vi "simulation_to_image.vi"() -> (3 "Image Out":T1)   [LabVIEW 2010]
uses:
  <vilib>/vision/Image Controls.llb/IMAQ Image.ctl
  simulation_globals.vi
  red_tweezers_globals_INTERNAL.vi
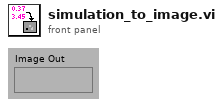
[diagram p1: front panel]
types:
  T1 = typedef "IMAQ Image.ctl" = refnum<image>
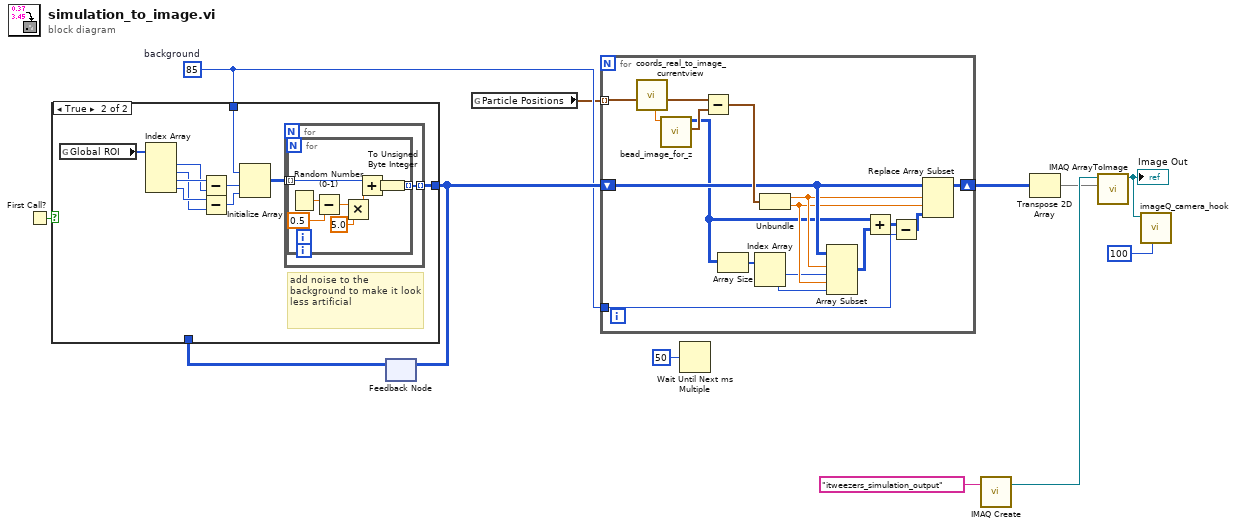
[diagram p0: block diagram]
diagram:
  w7 = u8 85  # background
  n1 = First Call?() -> (First Call?: T/F=w9:bool)
  n2 = feedback #1() -> (w10:u8[][])  [unwired: 1 in]
  n3 = case shown="True" w9 {
    tunnel: [w13 w15] -> w8
    tunnel: w10 -> [w13 _]
    tunnel: w7 -> [_ w14]
    frame False {
    }
    frame True {
      # "add noise to the background to make it look less artificial"
      n4 = global read "red_tweezers_globals_INTERNAL.vi" "Global ROI"() -> (w23:i32[])
      n5 = Index Array(array=w23) -> (element #1=w21:i32, element #2=w19:i32, element #3=w22:i32, element #4=w20:i32)  [unwired: 4 in]
      n6 = Subtract(x=w22, y=w21) -> (x-y=w18:i32)
      n7 = Subtract(x=w20, y=w19) -> (x-y=w17:i32)
      n8 = Initialize Array(w14, w18, w17) -> (w16:u8[][])
      n9 = for {
        tunnel: w16 -> [w25] mode=indexing
        tunnel: [w24] -> w15 mode=indexing
        n10 = for {
          tunnel: w25 -> [w28] mode=indexing
          tunnel: [w26] -> w24 mode=indexing
          n11 = Random Number (0-1)() -> (number: 0 to 1=w33:dbl)
          n12 = Subtract(x=w33, y=0.5) -> (x-y=w31:dbl)
          n13 = Multiply(x=w31, y=5.0) -> (x*y=w29:dbl)
          n14 = Add(x=w28, y=w29) -> (x+y=w27:dbl)
          n15 = To Unsigned Byte Integer(number=w27) -> (unsigned 8bit integer=w26:u8)
        }
      }
    }
  }
  n16 = feedback-in #1(w8) -> ()
  n17 = global read "simulation_globals.vi" "Particle Positions"() -> (w6:cluster{dbl, dbl, dbl}[])
  n18 = for {
    tunnel: w6 -> [w50] mode=indexing
    shift-right: [w47] -> w4
    shift-left: w8 -> [w44]
    tunnel: w7 -> [w34]
    n19 = call "coords_real_to_image_currentview.vi"("Position (real coords)"=w50) -> ("Position (pixels, relative to the top left of the image)"=w49:cluster{dbl, dbl}, "z (real coords)"=w46:dbl)  [unwired: 7 in]
    n20 = call "bead_image_for_z.vi"("Z/m"=w46) -> ("centre position"=w45:cluster{"[0]":dbl, "[1]":dbl}, "Image as U8 array"=w38:u8[][])  [unwired: 9 in]
    n21 = Subtract(x=w49, y=w45) -> (x-y=w48:cluster{dbl, dbl})
    n22 = Array Size(array=w38) -> (size(s)=w41:i32[])
    n23 = Index Array(array=w41) -> (element #1=w40:i32, element #2=w39:i32)  [unwired: 2 in]
    n24 = Unbundle(w48) -> (w43:dbl, w42:dbl)
    n25 = Array Subset(array=w44, index (row)=w43, length (row)=w40, index (col)=w42, length (col)=w39) -> (w37:u8[][])
    n26 = Add(x=w38, y=w37) -> (x+y=w35:u8[][])
    n27 = Subtract(x=w35, y=w34) -> (x-y=w36:u8[][])
    n28 = Replace Array Subset(array=w44, new element=w36, index (row)=w43, index (col)=w42) -> (w47:u8[][])
  }
  n29 = Wait Until Next ms Multiple(millisecond multiple=u32 50) -> ()  [unwired: 1 out]
  n30 = call "IMAQ Create"("Image Name"="itweezers_simulation_output") -> ("New Image"=w11:T1)  [unwired: 4 in, 1 out]
  n31 = Transpose 2D Array(2D array=w4) -> (transposed array=w2:u8[][])
  n32 = call "IMAQ ArrayToImage"("Image Pixels (U8)"=w2, "Image"=w11) -> ("Image Out"=w3:T1)  [unwired: 8 in, 1 out]
  "Image Out" <- w3
  n33 = call "imageQ_camera_hook.vi"("timeout in ms (0=don't wait if there are no requests)"=100, "Image"=w3) -> ()  [unwired: 10 in]
